vi "serial_write.vi"(0 "FPGA I/O In":refnum<k21>="RMC/DIO0", 5 "Serial write 1":u8[](array[numeric])=[0, 0, 0, 0, 0, 0, 0, 0, 0, 0, 0, 0, 0, 0, 0, 0, 0, 0, 0, 0, 0, 0, 0, 0, 0, 0, 0, 0, 0, 0, 0, 0, 0, 0, 0, 0, 0, 0, 0, 0, 0, 0, 0, 0, 0, 0, 0, 0, 0, 0, 0, 0, 0, 0, 0, 0, 0, 0, 0, 0, 0, 0, 0, 0, 0, 0, 0, 0, 0, 0, 0, 0, 0, 0, 0, 0, 0, 0, 0, 0, 0, 0, 0, 0, 0, 0, 0, 0, 0, 0, 0, 0, 0, 0, 0, 0, 0, 0, 0, 0], 7 "byte to write":i32, 9 "tick every bit":u32, 11 "tick after stop bit":u32) -> ()   [LabVIEW 2012]
uses:
  <vilib>/rvi/eio/common/nirviEmuTemplateMethod_errors.vi
  <vilib>/eio/EIONode/EIONode.xnode
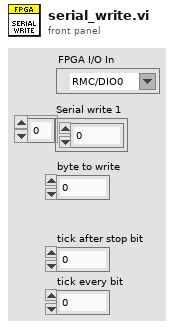
[diagram p1: front panel]
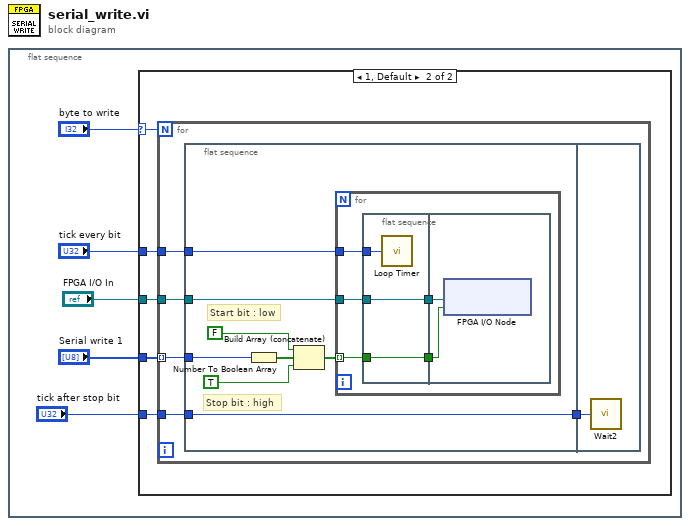
[diagram p0: block diagram]
diagram:
  n1 = flat-sequence {
    frame #0 {
      n2 = case shown="1, Default" "byte to write" {
        selector: "byte to write" -> [_ w10]
        tunnel: "FPGA I/O In" -> [_ w9]
        tunnel: "tick every bit" -> [_ w8]
        tunnel: "tick after stop bit" -> [_ w7]
        tunnel: "Serial write 1" -> [_ w6]
        frame 0 {
        }
        frame 1, Default {
          n3 = for {
            N: w10 -> [_]
            tunnel: w9 -> [w15]
            tunnel: w8 -> [w14]
            tunnel: w7 -> [w12]
            tunnel: w6 -> [w11] mode=indexing
            n4 = flat-sequence {
              tunnel: [w17] -> w13
              tunnel: w11 -> [w16]
              tunnel: w12 -> [w17]
              tunnel: w14 -> [w18]
              tunnel: w15 -> [w23]
              tunnel: w13 -> [w34]
              frame #0 {
                # "Start bit : low"
                # "Stop bit : high"
                n5 = Number To Boolean Array(number=w16) -> (Boolean array=w22:bool[])
                n6 = Build Array (concatenate)(FALSE, w22, TRUE) -> (w19:bool[])
                n7 = for {
                  tunnel: w19 -> [w28] mode=indexing
                  tunnel: w23 -> [w27]
                  tunnel: w18 -> [w24]
                  n8 = flat-sequence {
                    tunnel: w27 -> [w30]
                    tunnel: w28 -> [w31]
                    tunnel: [w31] -> w26
                    tunnel: [w30] -> w25
                    tunnel: w24 -> [w29]
                    tunnel: w26 -> [w33]
                    tunnel: w25 -> [w32]
                    frame #0 {
                      n9 = call "Loop Timer"("Count(Ticks)"=w29) -> ()  [unwired: 1 out]
                    }
                    frame #1 {
                      n10 = xnode "FPGA I/O Node"("I/O Item"=w33, "FPGA I/O In"=w32) -> ()  [unwired: 1 out]
                    }
                  }
                }
              }
              frame #1 {
                n11 = call "Wait2"("Count(Ticks)"=w34) -> ()  [unwired: 1 out]
              }
            }
          }
        }
      }
    }
  }
